vi "sub_vi_arduino_communication.vi"(5 "Cycles":i32, 6 "error in (no error)":errorcluster, 7 "write buffer":string, 8 "Function":i32, 9 "VISA resource name in":refnum<visa-resource-name>) -> (0 "error out":errorcluster, 1 "Reads array":dbl[](array[numeric]), 3 "VISA resource name out":refnum<visa-resource-name>, 4 "Received data":string[][](array[string]))   [LabVIEW 2019]
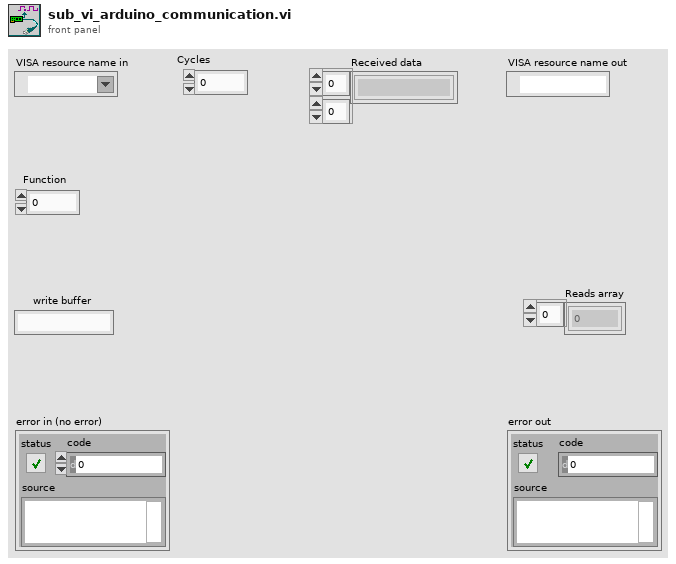
[diagram p1: front panel]
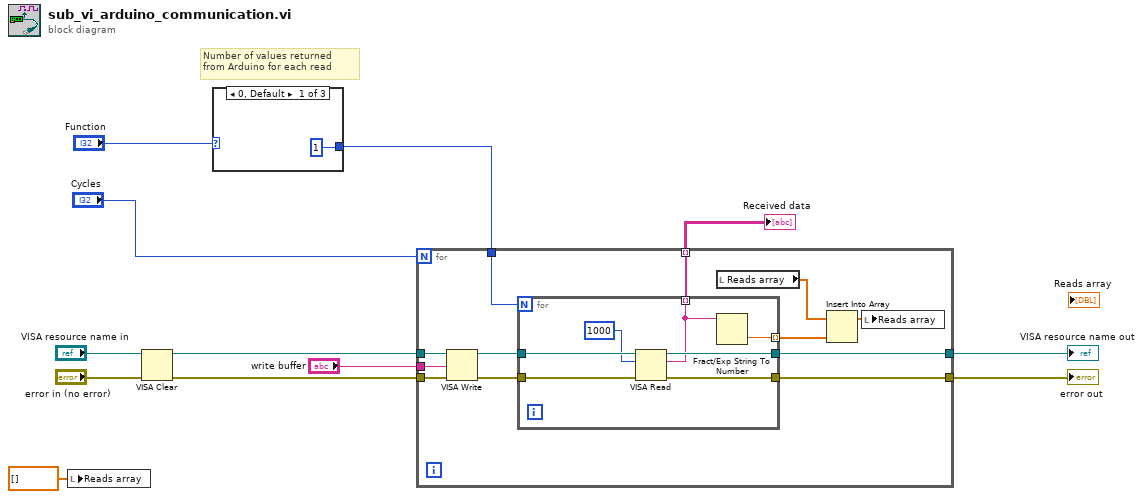
[diagram p0: block diagram]
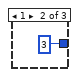
[diagram p2: hidden frame]
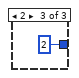
[diagram p3: hidden frame]
diagram:
  # "Number of values returned \nfrom Arduino for each read"
  n1 = local write "Reads array"(dbl[] [] ("Reads array")) -> ()
  n2 = VISA Clear(VISA resource name="VISA resource name in", error in (no error)="error in (no error)") -> (VISA resource name out=w8:refnum<visa-resource-name>, error out=w6:errorcluster)
  n3 = case shown="0, Default" "Function" {
    tunnel: [1 3 2] -> w3
    frame 0, Default {
    }
    frame 1 {
    }
    frame 2 {
    }
  }
  n4 = for {
    N: "Cycles" -> [_]
    tunnel: "write buffer" -> [w25]
    tunnel: w6 -> [w23]
    tunnel: [w27] -> w12
    tunnel: w8 -> [w24]
    tunnel: [w26] -> w11
    tunnel: w3 -> [w20]
    tunnel: [w19] -> w2 mode=indexing
    n5 = VISA Write(VISA resource name=w24, write buffer=w25, error in (no error)=w23) -> (VISA resource name out=w21:refnum<visa-resource-name>, error out=w22:errorcluster)  [unwired: 1 out]
    n6 = for {
      N: w20 -> [_]
      tunnel: w21 -> [w31]
      tunnel: [w33] -> w26
      tunnel: w22 -> [w32]
      tunnel: [w34] -> w27
      tunnel: [w29] -> w19 mode=indexing
      tunnel: [w28] -> w18 mode=indexing
      n7 = VISA Read(VISA resource name=w31, byte count=u32 1000, error in (no error)=w32) -> (VISA resource name out=w33:refnum<visa-resource-name>, read buffer=w29:string, error out=w34:errorcluster)  [unwired: 1 out]
      n8 = Fract/Exp String To Number(string=w29) -> (number=w28:dbl)  [unwired: 3 in, 1 out]
    }
    n9 = local read "Reads array"() -> (w17:dbl[])
    n10 = Insert Into Array(array=w17, new element=w18) -> (w16:dbl[])  [unwired: 1 in]
    n11 = local write "Reads array"(w16) -> ()
  }
  "error out" <- w12
  "VISA resource name out" <- w11
  "Received data" <- w2
